vi "End Scanning Trial.vi"(8 "error in (no error)":errorcluster, 11 "NI Force Task in":refnum<class "NI Force Task.lvclass">) -> (0 "error out":errorcluster, 3 "NI Force Task out":refnum<class "NI Force Task.lvclass">)   [LabVIEW 2020, in "NI Force Task.lvlib" / "NI Force Task.lvclass"]
uses:
  NI Force Task.lvclass
  NI Force Task.lvclass/NI Force Task.ctl
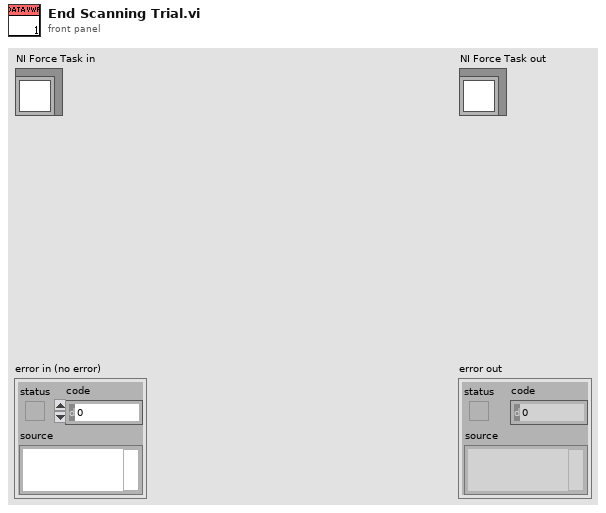
[diagram p1: front panel]
types:
  T1 = typedef "Task info df.ctl" = cluster{"Number of Trials":u8, "Sampling Rate (Hz)":u16, "Trial Duration (s)":u8, "Adjusted MVC (N)":dbl, "R Phase":i32, "L Phase":i32, "L Pattern":u8, "R Pattern":u8, "Time Between Trials (s)":u8, "Lissajous Speed":u16}
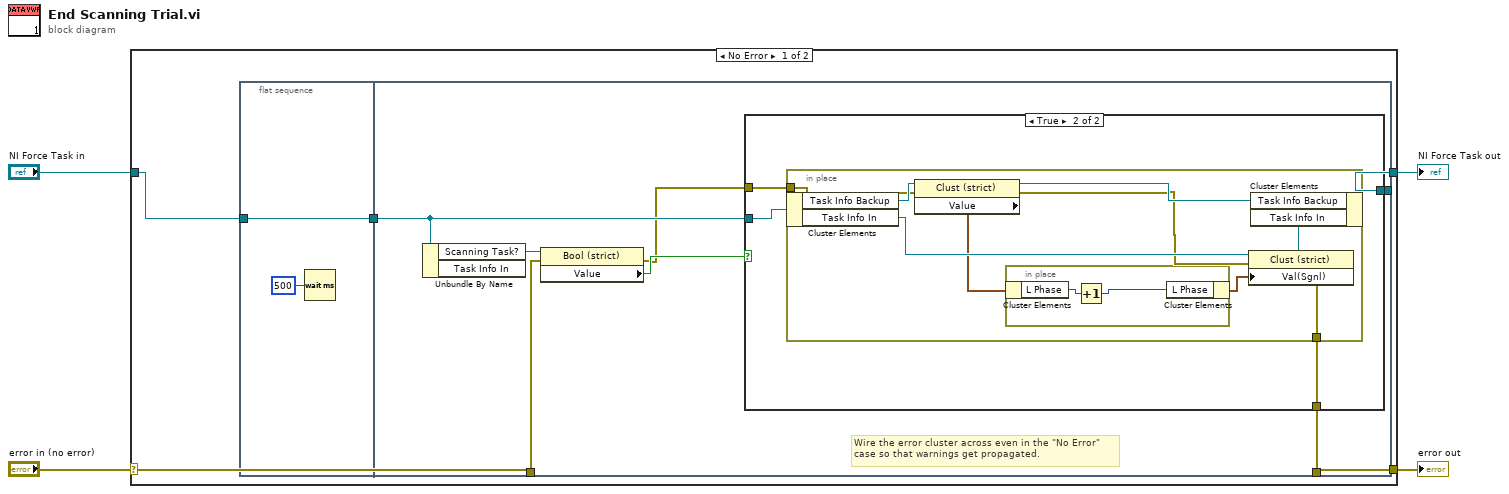
[diagram p0: block diagram]
diagram:
  n1 = case shown="No Error" "error in (no error)" {
    selector: "error in (no error)" -> [w7 w37]
    tunnel: [w6 w37] -> w3
    tunnel: [w9 w36] -> w1
    tunnel: "NI Force Task in" -> [w8 w36]
    frame No Error {
      n2 = flat-sequence {
        tunnel: w8 -> [w11]
        tunnel: [w11] -> w5
        tunnel: [w18] -> w9
        tunnel: w7 -> [w14]
        tunnel: [w12] -> w6
        tunnel: w5 -> [w17]
        frame #0 {
          n3 = Wait (ms)(milliseconds to wait=u32 500) -> ()  [unwired: 1 out]
        }
        frame #1 {
          # "Wire the error cluster across even in the \"No Error\"\ncase so that warnings get propagated."
          n4 = Unbundle By Name(w17) -> ("Scanning Task?"=w16:refnum<vi>)  [unwired: 1 out]
          n5 = property class="Bool (strict)"(reference=w16, error in=w14) -> (error out=w13:errorcluster, "Value"=w15:bool)  [unwired: 1 out]
          n6 = case shown="True" w15 {
            tunnel: [w20 w24] -> w18
            tunnel: w17 -> [w20 w23]
            tunnel: w13 -> [w19 w22]
            tunnel: [w19 w21] -> w12
            frame False {
            }
            frame True {
              n7 = in-place {
                in-place-border: w22 -> [w29]
                in-place-border: [w27] -> w21
                n8 = in-place-cluster #1(w23) -> ("Task Info Backup"=w32:refnum<vi>, "Task Info In"=w30:refnum<vi>)
                n9 = property class="Clust (strict)"(reference=w32, error in=w29) -> (reference out=w31:refnum<vi>, error out=w28:errorcluster, "Value"=w26:T1)
                n10 = in-place {
                  n11 = in-place-cluster #2(w26) -> ("L Phase"=w35:i32)
                  n12 = Increment(x=w35) -> (x+1=w34:i32)
                  n13 = in-place-cluster #2("L Phase"=w34) -> (w25:T1)
                }
                n14 = property class="Clust (strict)"(reference=w30, error in=w28, "Val(Sgnl)"=w25) -> (reference out=w33:refnum<vi>, error out=w27:errorcluster)
                n15 = in-place-cluster #1("Task Info Backup"=w31, "Task Info In"=w33) -> (w24:refnum<class "NI Force Task.lvclass">)
              }
            }
          }
        }
      }
    }
    frame Error {
    }
  }
  "error out" <- w3
  "NI Force Task out" <- w1
